vi "改变列宽.vi"(10 "列数":i32, 11 "引用":refnum<vi>) -> ()   [LabVIEW 8.6]
uses:
  <vilib>/Utility/miscctls.llb/LVRowAndColumnTypeDef.ctl
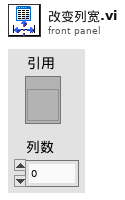
[diagram p1: front panel]
types:
  T1 = typedef "LVRowAndColumnTypeDef.ctl" = cluster{"Row":i32, "Column":i32}
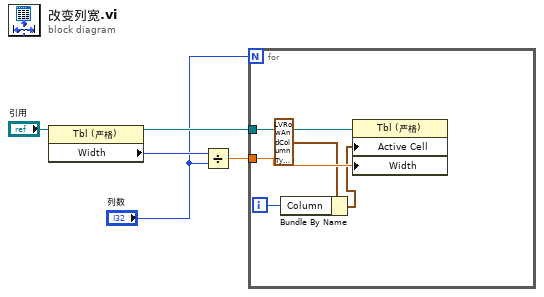
[diagram p0: block diagram]
diagram:
  n1 = property class="Tbl (严格)"(reference="引用") -> (reference out=w4:refnum<vi>, "Width"=w5:u32)  [unwired: 1 in, 1 out]
  n2 = Divide(x=w5, y="列数") -> (x/y=w2:dbl)
  n3 = for {
    N: "列数" -> [_]
    tunnel: w4 -> [w10]
    tunnel: w2 -> [w9]
    i -> [w7]
    n4 = Bundle By Name(cluster=T1 ? ("活动单元格:活动单元格"), "Column"=w7) -> (w6:T1)
    n5 = property class="Tbl (严格)"(reference=w10, "Active Cell"=w6, "Width"=w9) -> ()  [unwired: 1 in, 2 out]
  }
